vi "ArmLower.vi"() -> ()   [LabVIEW 2018]
panel:
  in  "ArmLower":bool
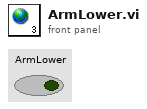
[diagram p1: front panel]
diagram:
